vi "Write Local OOB Data.vi"(8 "error in":errorcluster, 10 "Local OOB Data":variant, 11 "OOB in":refnum<class "CIFOutOfBand.lvclass">) -> (0 "error out":errorcluster, 3 "OOB out":refnum<class "CIFOutOfBand.lvclass">)   [LabVIEW 2021, in "CIFOutOfBand.lvclass"]
uses:
  CIFOutOfBand.lvclass
  CIFOutOfBand.lvclass/CIFOutOfBand.ctl
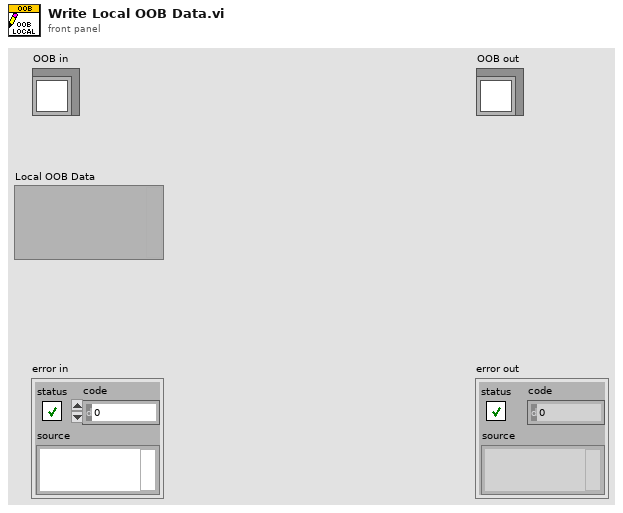
[diagram p1: front panel]
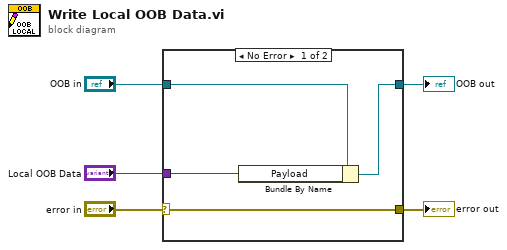
[diagram p0: block diagram]
diagram:
  n1 = case shown="No Error" "error in" {
    selector: "error in" -> [w9 w10]
    tunnel: [w9 w10] -> w4
    tunnel: [w7 w11] -> w2
    tunnel: "OOB in" -> [w8 w11]
    tunnel: "Local OOB Data" -> [w6 _]
    frame No Error {
      n2 = Bundle By Name(cluster=w8, "Payload"=w6) -> (w7:refnum<class "CIFOutOfBand.lvclass">)
    }
    frame Error {
    }
  }
  "error out" <- w4
  "OOB out" <- w2
